vi "Add Control to Server ClusterDef.vi"(5 "New Control Label":string, 6 "Clear Previous ?(T)":bool=TRUE, 7 "Source Control ref in":refnum<vi>, 8 "error in (no error)":errorcluster, 10 "Target ClusterDef Name":string, 11 "Server class in":refnum<vi>) -> (0 "error out":errorcluster, 3 "Server class out":refnum<vi>)   [LabVIEW 2019, in "gRPC Scripting Tools.lvlib"]
uses:
  gRPC Scripting Tools.lvlib
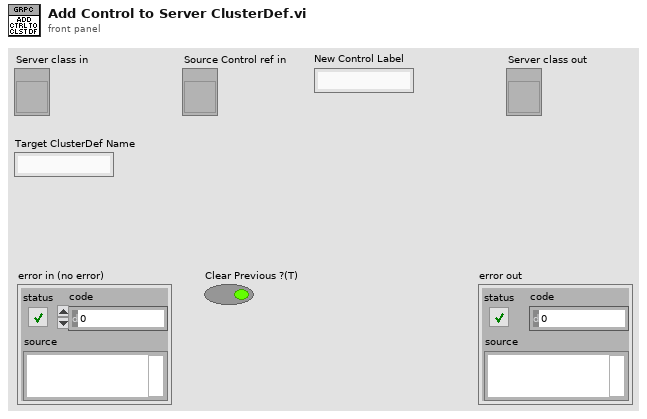
[diagram p1: front panel]
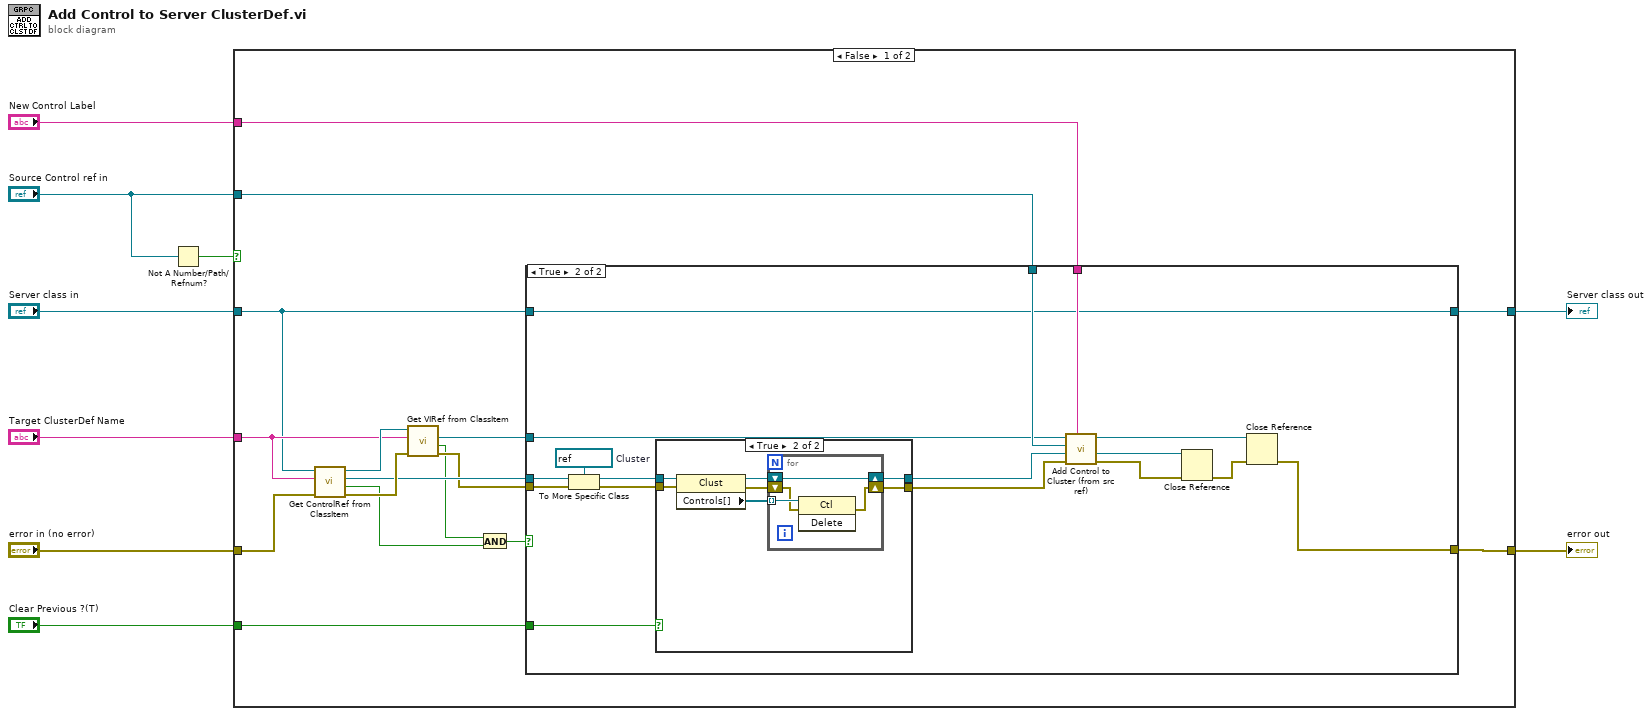
[diagram p0: block diagram]
diagram:
  n1 = Not A Number/Path/Refnum?(number/path/refnum="Source Control ref in") -> (NaN/Path/Refnum?=w1:bool)
  n2 = case shown="False" w1 {
    tunnel: [w25 w58] -> w9
    tunnel: "Target ClusterDef Name" -> [w22 _]
    tunnel: "error in (no error)" -> [w19 w58]
    tunnel: "New Control Label" -> [w18 _]
    tunnel: "Server class in" -> [w13 w59]
    tunnel: [w12 w59] -> w4
    tunnel: "Clear Previous ?(T)" -> [w11 _]
    tunnel: "Source Control ref in" -> [w10 _]
    frame False {
      n3 = call "Get ControlRef from ClassItem.vi"("error in (no error)"=w19, "Item Name"=w22, "LVClassLibrary in"=w13) -> ("error out"=w21:errorcluster, "Found ?"=w16:bool, "Control ref out"=w20:refnum<vi>, "LVClassLibrary out"=w23:refnum<vi>)  [unwired: 5 in]
      n4 = call "Get VIRef from ClassItem.vi"("error in (no error)"=w21, "Item Name"=w22, "LVClassLibrary in"=w23) -> ("error out"=w17:errorcluster, "Found ?"=w15:bool, "VIref out"=w24:refnum<vi>)  [unwired: 5 in, 1 out]
      n5 = And(x=w15, y=w16) -> (x .and. y?=w14:bool)
      n6 = case shown="True" w14 {
        tunnel: [w26 w44] -> w25
        tunnel: w10 -> [_ w41]
        tunnel: w24 -> [_ w40]
        tunnel: w20 -> [_ w38]
        tunnel: w18 -> [_ w36]
        tunnel: w17 -> [w26 w35]
        tunnel: w13 -> [w27 w34]
        tunnel: [w27 w34] -> w12
        tunnel: w11 -> [_ w29]
        frame False {
          # "#TODO Generate an error here?"
        }
        frame True {
          w37 = refnum<vi> refnum  # Cluster
          n7 = To More Specific Class(target class=w37, reference=w38, error in=w35) -> (specific class reference=w33:refnum<vi>, error out=w32:errorcluster)
          n8 = case shown="True" w29 {
            tunnel: w33 -> [w46 w53]
            tunnel: w32 -> [w45 w52]
            tunnel: [w46 w49] -> w31
            tunnel: [w45 w47] -> w30
            frame False {
            }
            frame True {
              n9 = property class="Clust"(reference=w53, error in=w52) -> (reference out=w50:refnum<vi>, error out=w48:errorcluster, "Controls[]"=w51:refnum<vi>[])
              n10 = for {
                tunnel: w51 -> [w57] mode=indexing
                shift-right: [w56] -> w49
                shift-left: w50 -> [w56]
                shift-right: [w54] -> w47
                shift-left: w48 -> [w55]
                n11 = invoke class="Ctl" method="Delete"(reference=w57, error in=w55) -> (error out=w54:errorcluster)  [unwired: 1 in, 2 out]
              }
            }
          }
          n12 = call "Add Control to Cluster (from src ref).vi"("New Control Label"=w36, "error in (no error)"=w30, "Cluster ref in (owner)"=w31, "Control ref in"=w41, "Owning VI ref in"=w40) -> ("error out"=w39:errorcluster, "Cluster ref out (owner)"=w42:refnum<vi>, "Owning VI ref out"=w43:refnum<vi>)  [unwired: 3 in, 1 out]
          n13 = Close Reference(reference=w42, error in (no error)=w39) -> (error out=w28:errorcluster)
          n14 = Close Reference(reference=w43, error in (no error)=w28) -> (error out=w44:errorcluster)
        }
      }
    }
    frame True {
    }
  }
  "error out" <- w9
  "Server class out" <- w4
